vi "周期设置_多参数.vi"() -> ()   [LabVIEW 2016, in "斯坦道多参数.lvlib"]
uses:
  <vilib>/Utility/miscctls.llb/LVPointTypeDef.ctl
  <vilib>/ptbypt/NI_PtbyPt.lvlib
  <vilib>/Utility/config.llb/NI_LVConfig.lvlib
panel:
  in  "运行周期":T1
  # "运行模式："
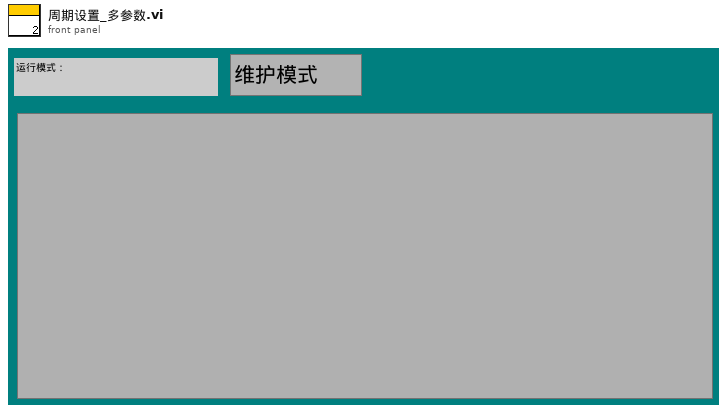
[diagram p1: front panel]
types:
  T1 = cluster{"运行模式":enum16{"维护模式", "常规模式", "应急模式", "质控模式"}, "24H周期设置":bool[]}
  T2 = typedef "LVPointTypeDef.ctl" = cluster{"Horizontal":i16, "Vertical":i16}
  T3 = typedef "LVDateTimeRec.ctl" = cluster{"秒数的小数部分":dbl, "秒":i32, "分":i32, "时":i32, "日":i32, "月":i32, "年":i32, "天数（周）":i32, "天数（年）":i32, "DST":i32}
  T4 = enum32{"Bad", "Idle", "Run top level", "Running"}
  T5 = typedef "NI_LVConfig.lvlib/Config Data RefNum.ctl" = refnum<k1>
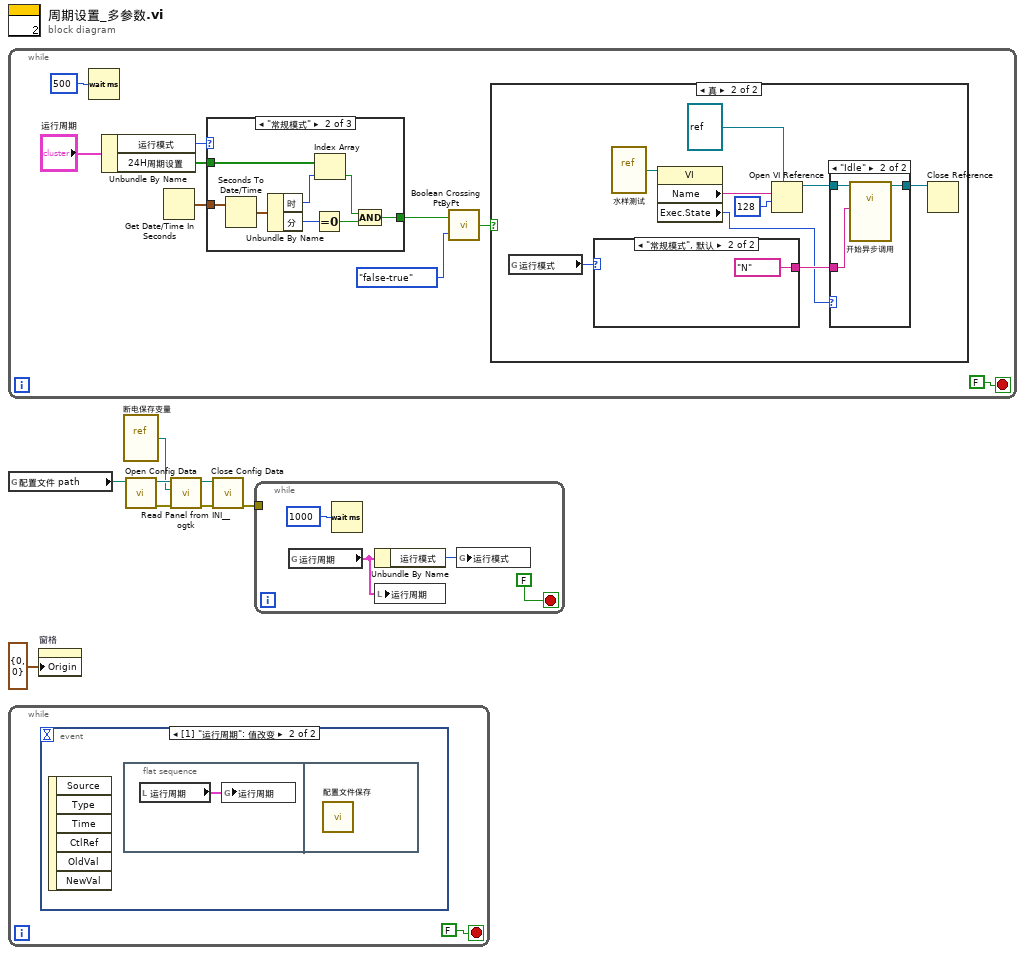
[diagram p0: block diagram]
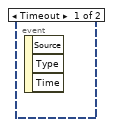
[diagram p2: hidden frame]
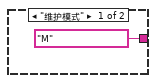
[diagram p4: hidden frame]
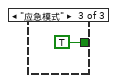
[diagram p7: hidden frame]
diagram:
  n1 = while {
    stop <- FALSE stop-if-true
    n2 = Wait (ms)(milliseconds to wait=u32 500 ("等待时间（毫秒）")) -> ()  [unwired: 1 out]
    n3 = Unbundle By Name("运行周期") -> ("运行模式"=w12:enum16{"维护模式", "常规模式", "应急模式", "质控模式"}, "24H周期设置"=w13:bool[])
    n4 = Get Date/Time In Seconds() -> (seconds since 1Jan1904=w17:timestamp)
    n5 = case shown="\"常规模式\"" w12 {
      tunnel: w17 -> [_ w40 _]
      tunnel: w13 -> [_ w37 _]
      tunnel: [_ w33 TRUE] -> w11
      frame "维护模式", Default {
      }
      frame "常规模式" {
        n6 = Seconds To Date/Time(time stamp (now)=w40) -> (date time rec=w39:T3)  [unwired: 1 in]
        n7 = Unbundle By Name(w39) -> ("时"=w38:i32, "分"=w36:i32)
        n8 = Equal To 0?(x=w36) -> (x = 0?=w34:bool)
        n9 = Index Array(array=w37, index=w38) -> (element=w35:bool)
        n10 = Compound Arithmetic op=AND ("复合运算")(w35, w34) -> (w33:bool)
      }
      frame "应急模式" {
      }
    }
    n11 = call <vilib>:"Boolean Crossing PtByPt.vi"("direction"=enum16{"either", "false-true", "true-false"}."false-true", "input"=w11) -> ("crossing"=w10:bool)  [unwired: 1 in]
    n12 = case shown="真" w10 {
      frame False {
      }
      frame True {
        n13 = global read "多参数全局变量.vi" "运行模式"() -> (w25:enum16{"维护模式", "常规模式", "应急模式", "质控模式"})
        n14 = case shown="\"常规模式\", 默认" w25 {
          tunnel: ["M" ("数据标记表") "N" ("数据标记表")] -> w26
          frame "维护模式" {
          }
          frame "常规模式", Default {
          }
        }
        n15 = vi-ref "水样测试.vi"() -> (w23:refnum<vi>)
        n16 = property class="VI"(reference=w23) -> ("Name"=w19:string, "Exec.State"=w21:T4)  [unwired: 1 in, 2 out]
        n17 = Open VI Reference(type specifier VI Refnum (for type only)=refnum<vi> refnum, vi path=w19, options=128 ("选项")) -> (vi reference=w18:refnum<vi>)  [unwired: 3 in, 1 out]
        n18 = case shown="\"Idle\"" w21 {
          tunnel: [w29 w32] -> w22
          tunnel: w18 -> [w29 w31]
          tunnel: w26 -> [_ w30]
          frame "Bad", Default {
          }
          frame "Idle" {
            n19 = call-by-ref "开始异步调用"(reference=w31, "数据标记表"=w30) -> (reference out=w32:refnum<vi>)  [unwired: 12 in, 1 out]
          }
        }
        n20 = Close Reference(reference=w22) -> ()  [unwired: 1 in, 1 out]
      }
    }
  }
  n21 = global read "多参数全局变量.vi" "配置文件 path"() -> (w2:path)
  n22 = while {
    stop <- FALSE stop-if-true
    n23 = event shown="[1] \"运行周期\": 值改变" {
      selector: _ -> [_ _]
      dyn-events: _ -> [_ _]
      timeout: _ -> [_ _]
      event Timeout {
        n24 = event-data() -> ()  [unwired: 1 in, 3 out]
      }
      event "运行周期": Value Change {
        n25 = event-data() -> ()  [unwired: 1 in, 6 out]
        n26 = flat-sequence {
          frame #0 {
            n27 = local read "运行周期"() -> (w43:T1)
            n28 = global write "断电保存变量.vi" "运行周期"(w43) -> ()
          }
          frame #1 {
            n29 = call "配置文件保存.vi"() -> ()  [unwired: 12 in]
          }
        }
      }
    }
  }
  n30 = property on="窗格" class="Pane"("Origin"=T2 {"Horizontal"=0, "Vertical"=0} ("原点")) -> ()  [unwired: 2 in, 2 out]
  n31 = vi-ref "断电保存变量.vi"() -> (w3:refnum<vi>)
  n32 = call <vilib>:"Open Config Data.vi"("configuration file path"=w2) -> ("error out"=w6:errorcluster, "refnum"=w7:T5)  [unwired: 8 in, 1 out]
  n33 = call <userlib>:"Read Panel from INI__ogtk.vi"("error in (no error)"=w6, "VI ref"=w3, "refnum"=w7) -> ("error out"=w4:errorcluster, "refnum out"=w5:T5)  [unwired: 7 in]
  n34 = call <vilib>:"Close Config Data.vi"("error in (no error)"=w4, "refnum"=w5) -> ("error out"=w1:errorcluster)  [unwired: 8 in, 1 out]
  n35 = while {
    tunnel: w1 -> [_]
    stop <- FALSE stop-if-true
    n36 = global read "断电保存变量.vi" "运行周期"() -> (w45:T1)
    n37 = Wait (ms)(milliseconds to wait=u32 1000 ("等待时间（毫秒）")) -> ()  [unwired: 1 out]
    n38 = Unbundle By Name(w45) -> ("运行模式"=w44:enum16{"维护模式", "常规模式", "应急模式", "质控模式"})
    n39 = local write "运行周期"(w45) -> ()
    n40 = global write "多参数全局变量.vi" "运行模式"(w44) -> ()
  }
